vi "AstromFalconGuinding.vi"() -> ()   [LabVIEW 2011]
panel:
  in  "Binning":u16(ring) items=["1 x 1"=1, "2 x 2"=2, "4 x 4"=4, "5 x 5"=5]
  in  "PIXSCALE":cluster{"pixscale2":dbl, "pixscale1":dbl}
  in  "NAXIS":cluster{"naxis2":u16, "naxis1":u16}
  in  "Dec Sonde":dbl=34150.89703708518 caption="DEC de la sonde" format="%<%H:%M:%S%0u>t"
  in  "RA Sonde":dbl=70407.2665759738 caption="RA de la sonde" format="%<%H:%M:%S%1u>t"
  in  "Rotation":dbl=133.394864 caption="Coupole" min=0.0 max=359.0 step=1.0
  out "Correction E-W":dbl
  out "Correction N-S":dbl
  out "Dec Reference":dbl=34150.93098198265 caption="Dec Cible" format="%<%H:%M:%S%0u>t"
  out "RA Reference":dbl=70407.26510530974 caption="RA de la Cible" format="%<%H:%M:%S%1u>t"
  out "Dec Centroid":dbl=34150.89703708518 caption="DEC de la sonde" format="%<%H:%M:%S%0u>t"
  out "RA Centroid":dbl=70407.2665759738 caption="RA de la sonde" format="%<%H:%M:%S%1u>t"
  in  "XReference":dbl caption="Pos" format="%.1f"
  in  "YReference":dbl caption="X          Y" format="%.1f"
  in  "XCentroid":dbl caption="Pos" format="%.1f"
  in  "YCentroid":dbl caption="X          Y" format="%.1f"
  out "GuiderAstrom":T1 {"CRVAL" format="%.6g"; "CD" format="%_7g"}
  # "RA"
  # "DEC"
  # "Sonde"
  # "RA"
  # "DEC"
  # "X"
  # "Y"
  # "Centroid"
  # "Reference"
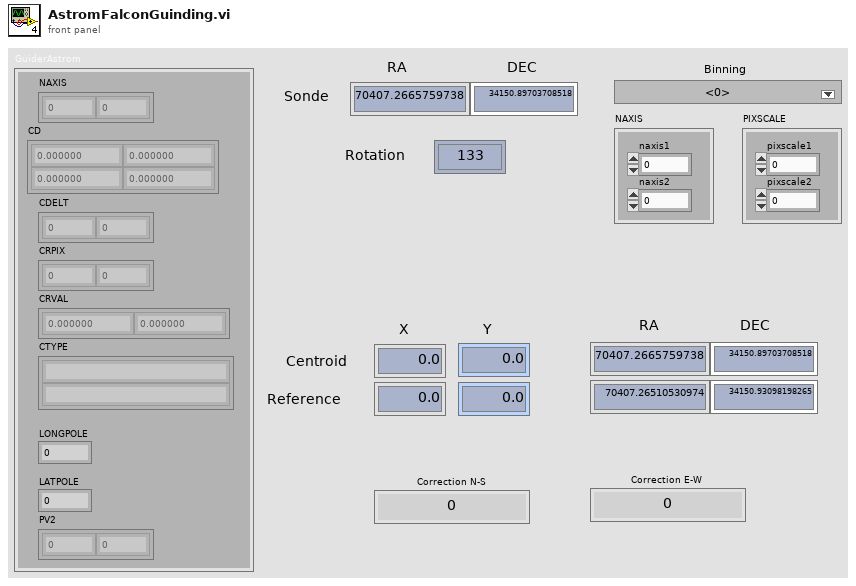
[diagram p1: front panel]
types:
  T1 = cluster{"NAXIS":dbl[], "CD":dbl[][], "CDELT":dbl[], "CRPIX":dbl[], "CTYPE":string[], "CRVAL":dbl[], "LONGPOLE":dbl, "LATPOLE":dbl, "PV2":dbl[]}
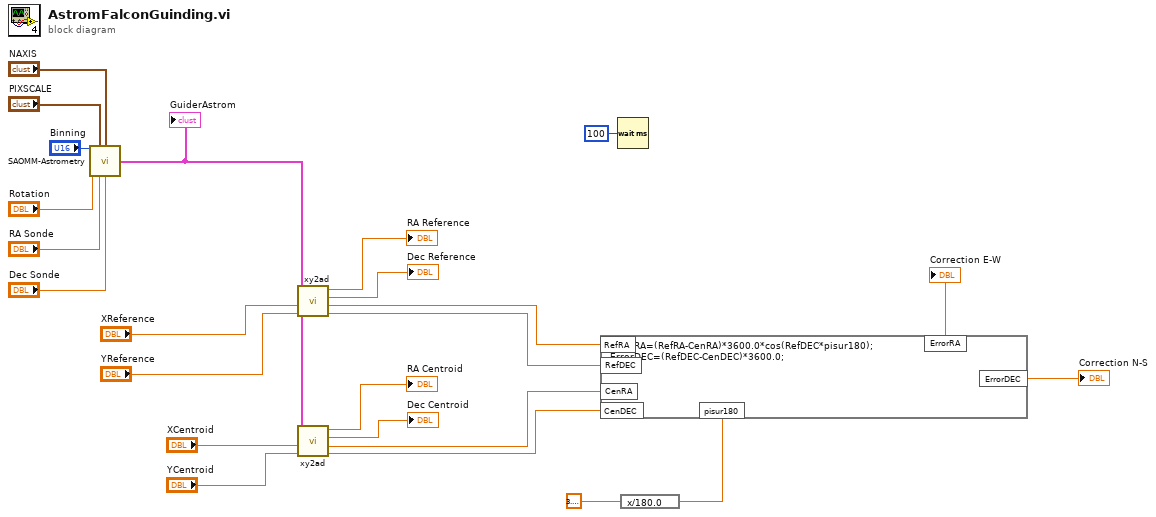
[diagram p0: block diagram]
diagram:
  n1 = call "SAOMM-Astrometry.vi"("Binning"="Binning", "PIXSCALE"="PIXSCALE", "NAXIS"="NAXIS", "Rotation"="Rotation", "RAsonde"="RA Sonde", "DECsonde"="Dec Sonde") -> ("GuideAstrom"=w18:T1)  [unwired: 9 in]
  "GuiderAstrom" <- w18
  n2 = call "xy2ad.vi"("Y (px)"="YReference", "X (px)"="XReference", "Astrometry"=w18) -> ("DEC (°)"=w14:dbl, "RA (°)"=w15:dbl, "DEC (HH:MM:SS)"=→"Dec Reference":dbl, "RA (HH:MM:SS.S)"=→"RA Reference":dbl)  [unwired: 5 in]
  n3 = call "xy2ad.vi"("Y (px)"="YCentroid", "X (px)"="XCentroid", "Astrometry"=w18) -> ("DEC (°)"=w17:dbl, "RA (°)"=w16:dbl, "DEC (HH:MM:SS)"=→"Dec Centroid":dbl, "RA (HH:MM:SS.S)"=→"RA Centroid":dbl)  [unwired: 5 in]
  n4 = Wait (ms)(milliseconds to wait=u32 100) -> ()  [unwired: 1 out]
  n5 = expression code="x/180.0"(3.141592653589793) -> (w9:dbl)
  n6 = formula code="ErrorRA=(RefRA-CenRA)*3600.0*cos(RefDEC*pisur180);\nErrorDEC=(RefDEC-CenDEC)*3600.0;"("RefRA"=w15, "RefDEC"=w14, "CenRA"=w16, "CenDEC"=w17, "pisur180"=w9) -> ("ErrorRA"=→"Correction E-W":dbl, "ErrorDEC"=→"Correction N-S":dbl)
